vi "Refocus Frame v6 with morphology selection.vi"() -> ()   [LabVIEW 2018]
uses:
  <vilib>/Analysis/NI_AALBase.lvlib
  <vilib>/vision/NI_Vision_Development_Module.lvlib
panel:
  out "Number of Particles":i32
  in  "Use size  filter?":bool
  in  "Selection Values":T2(array[cluster]) {"Measurement Parameter" items=["Center of Mass X", "Center of Mass Y", "First Pixel X", "First Pixel Y", "Bounding Rect Left", "Bounding Rect Top", "Bounding Rect Right", "Bounding Rect Bottom", "Max Feret Diameter Start X", "Max Feret Diameter Start Y", "Max Feret Diameter End X", "Max Feret Diameter End Y", "Max Horiz. Segment Length Left", "Max Horiz. Segment Length Right", "Max Horiz. Segment Length Row", "-", "Bounding Rect Width", "Bounding Rect Height", "Bounding Rect Diagonal", "Perimeter", "Convex Hull Perimeter", "Holes' Perimeter", "Max Feret Diameter", "Equivalent Ellipse Major Axis", "Equivalent Ellipse Minor Axis", "Equivalent Ellipse Minor Axis (Feret)", "Equivalent Rect Long Side", "Equivalent Rect Short Side", "Equivalent Rect Diagonal", "Equivalent Rect Short Side (Feret)", "Average Horiz. Segment Length", "Average Vert. Segment Length", "Hydraulic Radius", "Waddel Disk Diameter", "-", "Area", "Holes' Area", "Particle & Holes' Area", "Convex Hull Area", "Image Area", "-", "Number of Holes", "Number of Horiz. Segments", "Number of Vert. Segments", "-", "Orientation", "Max Feret Diameter Orientation", "-", "% Area/Image Area", "% Area/(Particle & Holes' Area)", "Ratio of Equivalent Ellipse Axes", "Ratio of Equivalent Rect Sides", "-", "Elongation Factor", "Compactness Factor", "Heywood Circularity Factor", "Type Factor", "-", "Sum X", "Sum Y", "Sum XX", "Sum XY", "Sum YY", "Sum XXX", "Sum XXY", "Sum XYY", "Sum YYY", "-", "Moment of Inertia XX", "Moment of Inertia XY", "Moment of Inertia YY", "Moment of Inertia XXX", "Moment of Inertia XXY", "Moment of Inertia XYY", "Moment of Inertia YYY", "Norm. Moment of Inertia XX", "Norm. Moment of Inertia XY", "Norm. Moment of Inertia YY", "Norm. Moment of Inertia XXX", "Norm. Moment of Inertia XXY", "Norm. Moment of Inertia XYY", "Norm. Moment of Inertia YYY", "Hu Moment 1", "Hu Moment 2", "Hu Moment 3", "Hu Moment 4", "Hu Moment 5", "Hu Moment 6", "Hu Moment 7"]; "Range Lower Value" format="%.2f"; "Range Upper Value" format="%.2f"}
  in  "Decimate by N\n(even number!)":i32=1
  in  "Use image file as background?\n(N=> calculate from movie input)":bool=TRUE
  in  "Background image":path
  in  "Brightness (default = 1)":dbl=1.0
  out "Image":T3(plugin-control)
  in  "Threshold":dbl
  in  "Set threshold":bool
  in  "Number of frames for median":u32=20
  in  "Read Frame Number":u32
  in  "Input Movie":path
  in  "# parallel loops":i32=12
  in  "Write Gradient stack?":bool
  in  "Write Refocused stack?":bool=TRUE
  in  "Flip Z-gradient?":bool
  in  "Bandpass Filter?":bool=TRUE
  in  "Smallest object (px)":dbl=2.0
  in  "Largest object (px)":dbl=30.0
  out "Currently calculating \nrefocused frame number:":i32
  in  "Medium refractive index":dbl=1.3326
  in  "Pixels/micron":dbl=0.711
  in  "Wavelength (um)":dbl=0.642
  in  "Step size (um)":dbl=10.0
  in  "Number of steps":i32=150
  in  "Start refocus value (um)":dbl
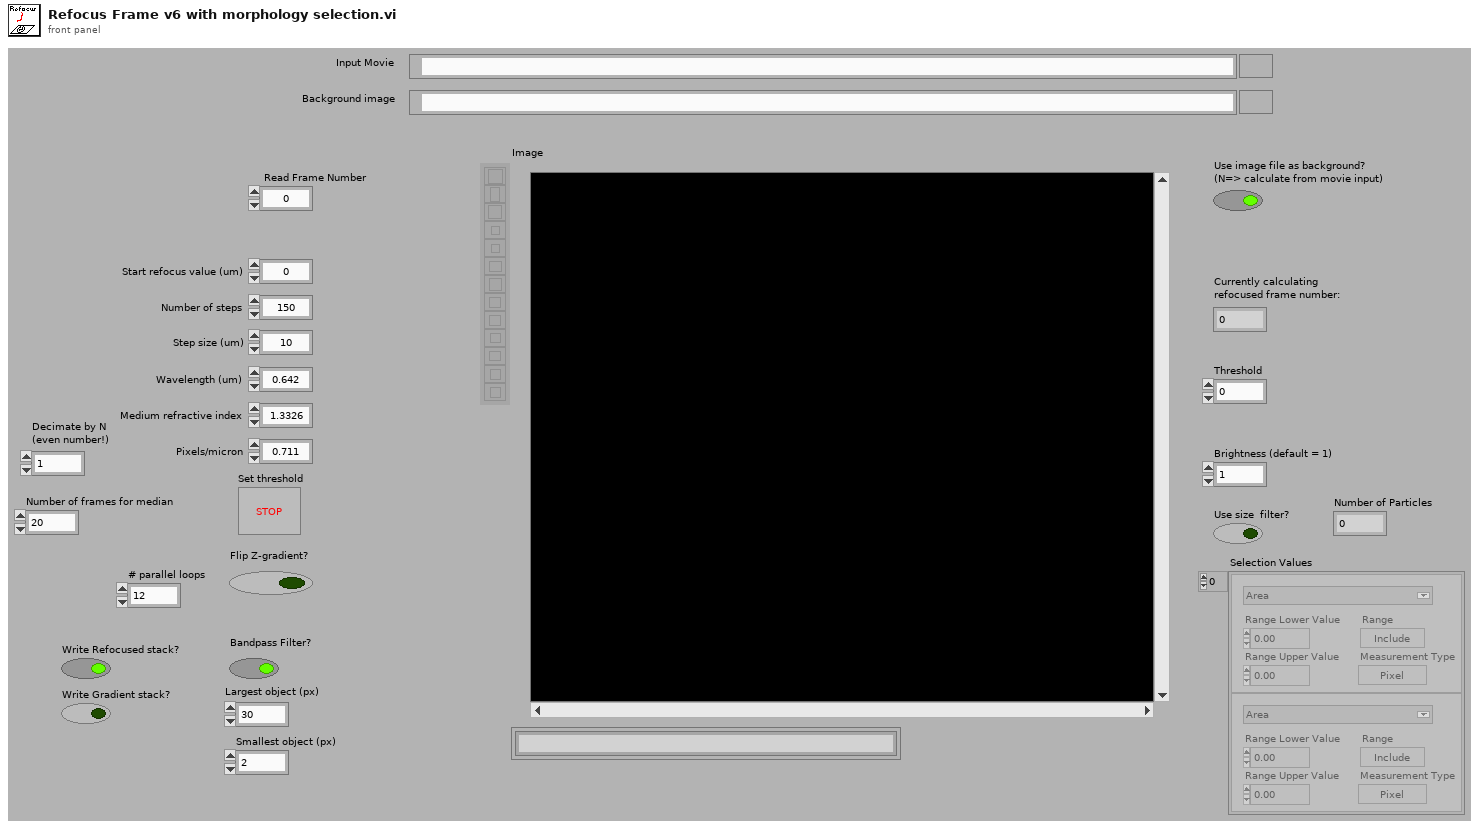
[diagram p1: front panel]
types:
  T1 = typedef "Particle Parameters" = i32
  T2 = cluster{"Measurement Parameter":T1, "Range Lower Value":dbl, "Range Upper Value":dbl, "Range":bool, "Measurement Type":bool}[]
  T3 = typedef "IMAQ Image.ctl" = refnum<image>
  T4 = typedef "Image Type" = u32
  T5 = typedef "AviRefnum.ctl" = refnum<k1>
  T6 = cluster{"Filter array":dbl[][], "Wavelength (um)":dbl, "Medium refractive index":dbl, dbl}
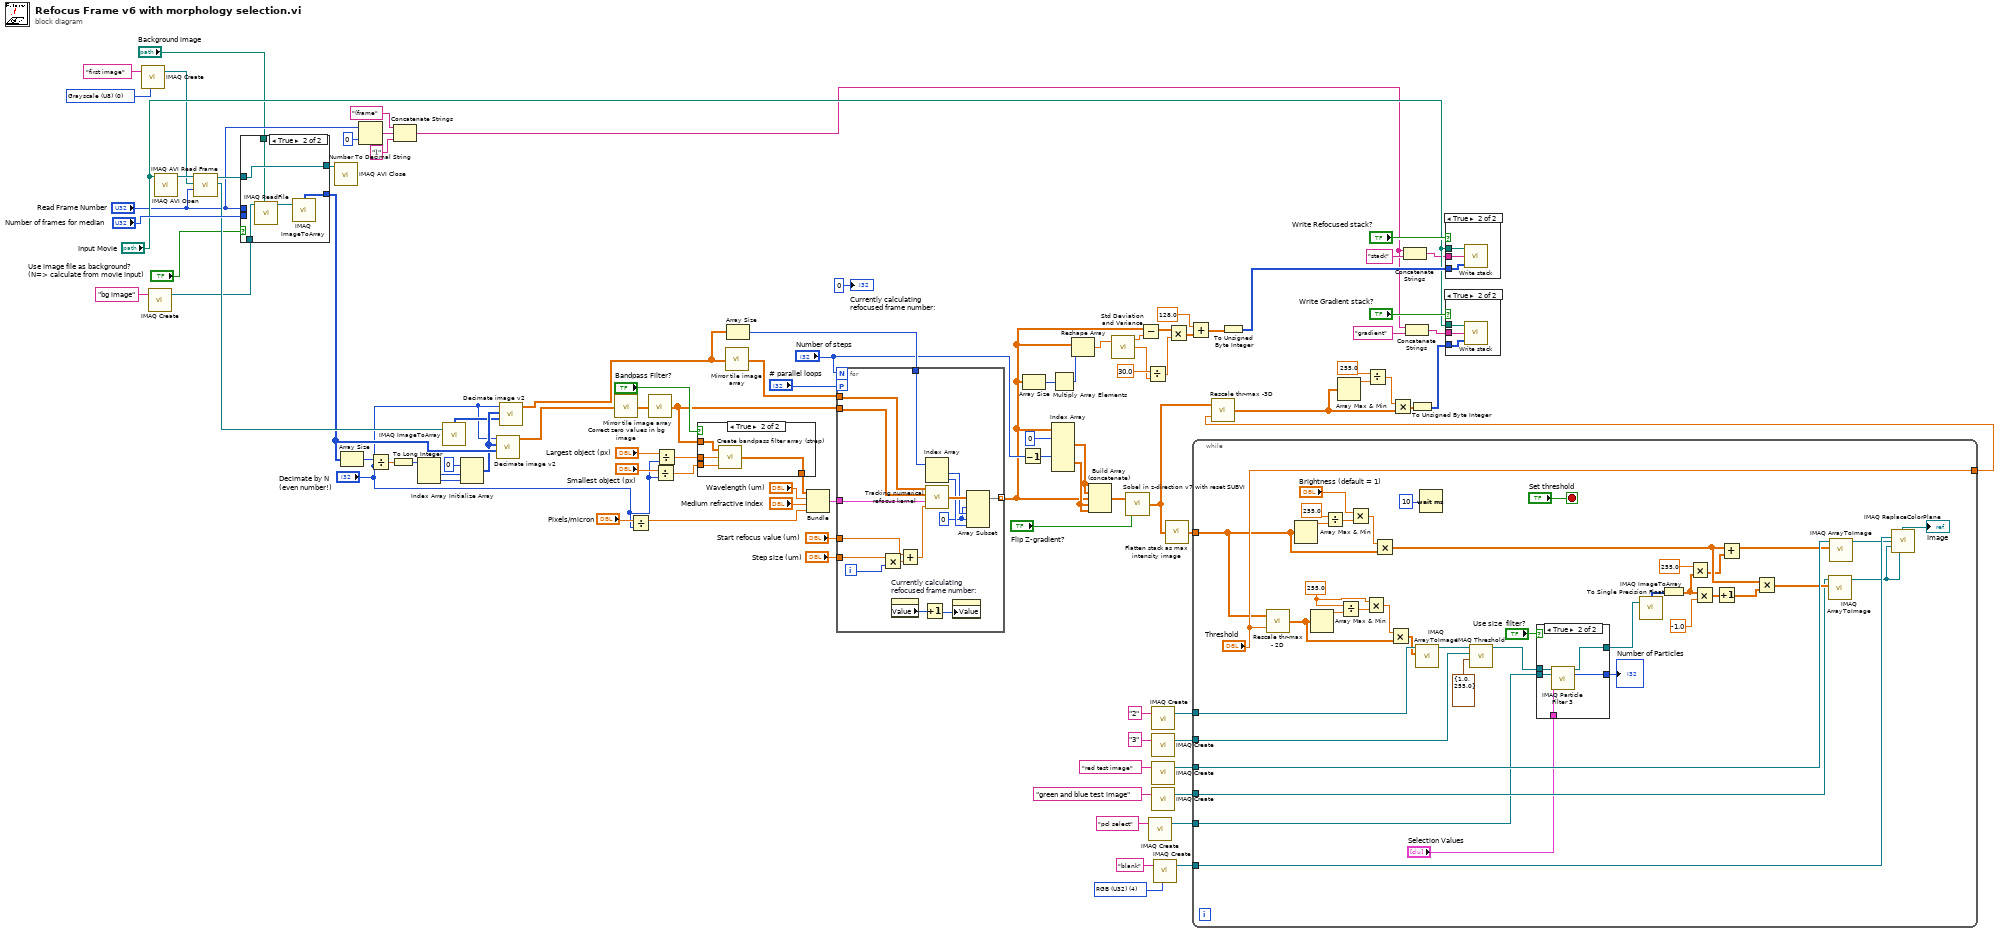
[diagram p0: block diagram]
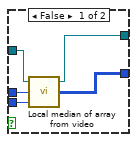
[diagram p2: hidden frame]
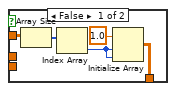
[diagram p6: hidden frame]
diagram:
  w3 = T4 4 items=["Grayscale (U8)", "Grayscale (I16)", "Grayscale (SGL)", "Complex (CSG)", "RGB (U32)", "HSL (U32)", "RGB (U64)", "Grayscale (U16)"] ("Image Type")
  w57 = T4 0 items=["Grayscale (U8)", "Grayscale (I16)", "Grayscale (SGL)", "Complex (CSG)", "RGB (U32)", "HSL (U32)", "RGB (U64)", "Grayscale (U16)"] ("Image Type")
  n1 = call "IMAQ Create"("Image Name"="first image", "Image Type"=w57) -> ("New Image"=w54:T3)  [unwired: 3 in, 1 out]
  n2 = call "IMAQ Create"("Image Name"="bg image") -> ("New Image"=w31:T3)  [unwired: 4 in, 1 out]
  n3 = call "IMAQ AVI Open"("AVI Path"="Input Movie") -> ("Avi Refnum"=w55:T5)  [unwired: 9 in, 1 out]
  n4 = call "IMAQ AVI Read Frame"("Frame Number"="Read Frame Number", "Image"=w54, "Avi Refnum"=w55) -> ("Image Out"=w53:T3, "Avi Refnum (duplicate)"=w52:T5)  [unwired: 5 in, 2 out]
  n5 = case shown="True" "Use image file as background?\n(N=> calculate from movie input)" {
    tunnel: "Number of frames for median" -> [w103 _]
    tunnel: w52 -> [w102 w108]
    tunnel: [w101 w108] -> w51
    tunnel: "Read Frame Number" -> [w100 _]
    tunnel: [w99 w104] -> w22
    tunnel: w31 -> [_ w106]
    tunnel: "Background image" -> [_ w105]
    frame False {
      n6 = call "Local median of array from video.vi"("Number of frames for median"=w103, "Read Frame Number"=w100, "Avi Refnum"=w102) -> ("Local median array"=w99:u8[][], "Avi Refnum (duplicate)"=w101:T5)  [unwired: 1 in]
    }
    frame True {
      n7 = call "IMAQ ReadFile"("File Path"=w105, "Image"=w106) -> ("Image Out"=w107:T3)  [unwired: 5 in, 4 out]
      n8 = call "IMAQ ImageToArray"("Image"=w107) -> ("Image Pixels (U8)"=w104:u8[][])  [unwired: 3 in, 4 out]
    }
  }
  n9 = call "IMAQ AVI Close"("Avi Refnum"=w51) -> ()  [unwired: 10 in, 1 out]
  n10 = Array Size(array=w22) -> (size(s)=w28:i32[])
  n11 = Number To Decimal String(number="Read Frame Number", width (-)=i16 0) -> (decimal integer string=w48:string)
  n12 = Divide(x=w28, y="Decimate by N\n(even number!)") -> (x/y=w27:dbl[])
  n13 = To Long Integer(number=w27) -> (32bit integer=w26:i32[])
  n14 = Concatenate Strings("(frame" ("string"), w48, ")" ("string")) -> (w42:string)
  n15 = Index Array(array=w26) -> (element #1=w25:i32, element #2=w24:i32)  [unwired: 2 in]
  n16 = call "IMAQ ImageToArray"("Image"=w53) -> ("Image Pixels (U8)"=w20:u8[][])  [unwired: 3 in, 4 out]
  n17 = Initialize Array(u8 0 ("element"), w25, w24) -> (w21:u8[][])
  n18 = call "Decimate image v2.vi"("Image Pixels (U8)"=w22, "Target array"=w21, "Decimate by N"="Decimate by N\n(even number!)") -> ("Filled target array"=w13:sgl[][])  [unwired: 8 in]
  n19 = call "Decimate image v2.vi"("Image Pixels (U8)"=w20, "Target array"=w21, "Decimate by N"="Decimate by N\n(even number!)") -> ("Filled target array"=w14:sgl[][])  [unwired: 8 in]
  n20 = call "Correct zero values in bg image.vi"("Image Pixels (U8)"=w13) -> ("Corrected array"=w83:sgl[][])
  n21 = Divide(x="Pixels/micron", y="Decimate by N\n(even number!)") -> (x/y=w19:dbl)
  n22 = call "Mirror tile image array.vi"("Image array"=w83) -> ("Mirror tiled array"=w81:sgl[][])
  n23 = Divide(x="Smallest object (px)", y="Decimate by N\n(even number!)") -> (x/y=w17:dbl)
  n24 = Divide(x="Largest object (px)", y="Decimate by N\n(even number!)") -> (x/y=w18:dbl)
  n25 = case shown="True" "Bandpass Filter?" {
    tunnel: w18 -> [_ w117]
    tunnel: w17 -> [_ w116]
    tunnel: w81 -> [w113 w115]
    tunnel: [w109 w114] -> w90
    frame False {
      n26 = Array Size(array=w113) -> (size(s)=w112:i32[])
      n27 = Index Array(array=w112) -> (element=w111:i32)  [unwired: 1 in]
      n28 = Initialize Array(1.0, w111, w111) -> (w109:dbl[][])
    }
    frame True {
      n29 = call "Create bandpass filter array (strep).vi"("Smallest object (pixels)"=w116, "Largest object (pixels)"=w117, "Image array"=w115) -> ("Filter array"=w114:dbl[][])
    }
  }
  n30 = call "Mirror tile image array.vi"("Image array"=w14) -> ("Mirror tiled array"=w84:sgl[][])
  n31 = Array Size(array=w14) -> (size(s)=w82:i32[])
  n32 = Bundle("Filter array"=w90, "Wavelength (um)"="Wavelength (um)", "Medium refractive index"="Medium refractive index", w19) -> (w92:T6)  [unwired: 1 in]
  n33 = for {
    N: "Number of steps" -> [_]
    tunnel: "Start refocus value (um)" -> [w131]
    tunnel: "Step size (um)" -> [w133]
    tunnel: w81 -> [w129]
    tunnel: [w125] -> w60 mode=indexing
    tunnel: w92 -> [w128]
    tunnel: w84 -> [w127]
    tunnel: w82 -> [w124]
    workers-P: "# parallel loops" -> [_]
    i -> [w120]
    w121 = 0 ("x+1")
    n34 = Multiply(x=w133, y=w120) -> (x*y=w132:dbl)
    n35 = property on="Currently calculating \nrefocused frame number:" class="DigNum (strict)"() -> ("Value"=w118:i32)  [unwired: 2 in, 2 out]
    n36 = Add(x=w131, y=w132) -> (x+y=w130:dbl)
    n37 = Increment(x=w118) -> (x+1=w119:i32)
    n38 = Index Array(array=w124) -> (element #1=w123:i32, element #2=w122:i32)  [unwired: 2 in]
    n39 = call "Tracking numerical refocus kernel.vi"("Defocus distance (um)"=w130, "Control Cluster"=w128, "Corrected array"=w129, "Image array"=w127) -> ("output array"=w126:dbl[][])
    n40 = property on="Currently calculating \nrefocused frame number:" class="DigNum (strict)"("Value"=w119) -> ()  [unwired: 2 in, 2 out]
    n41 = Array Subset(array=w126, index (row)=w121, length (row)=w123, index (col)=w121, length (col)=w122) -> (w125:dbl[][])
  }
  n42 = Decrement(x="Number of steps") -> (x-1=w74:i32)
  n43 = Array Size(array=w60) -> (size(s)=w61:i32[])
  n44 = Index Array(array=w60, index (dim 0) #1=0 ("x+1"), index (dim 0) #2=w74) -> (element #1=w73:dbl[][], element #2=w72:dbl[][])  [unwired: 4 in]
  n45 = Multiply Array Elements(1:w61) -> (0:w59:i32)
  n46 = Reshape Array(w60, w59) -> (w50:dbl[])
  n47 = Build Array (concatenate)(w73, w73, w60, w72, w72) -> (w71:dbl[][][])
  n48 = call <vilib>:"Std Deviation and Variance.vi"("X"=w50) -> ("mean"=w70:dbl, "standard deviation"=w68:dbl)  [unwired: 1 in, 1 out]
  n49 = call "Sobel in z-direction v7 with reset SUBVI.vi"("Flip Z-gradient?"="Flip Z-gradient?", "Recontructed Stack\n(with padded ends)"=w71) -> ("Sobel output stack"=w6:dbl[][][])
  n50 = Subtract(x=w60, y=w70) -> (x-y=w67:dbl[][][])
  n51 = Divide(x=30.0 ("Start refocus value (um)"), y=w68) -> (x/y=w66:dbl)
  n52 = call "IMAQ Create"("Image Name"="pcl select") -> ("New Image"=w1:T3)  [unwired: 4 in, 1 out]
  n53 = call "IMAQ Create"("Image Name"="2") -> ("New Image"=w11:T3)  [unwired: 4 in, 1 out]
  n54 = call "IMAQ Create"("Image Name"="3") -> ("New Image"=w9:T3)  [unwired: 4 in, 1 out]
  n55 = call "IMAQ Create"("Image Name"="red test image") -> ("New Image"=w38:T3)  [unwired: 4 in, 1 out]
  n56 = call "IMAQ Create"("Image Name"="green and blue test image") -> ("New Image"=w7:T3)  [unwired: 4 in, 1 out]
  n57 = call "IMAQ Create"("Image Name"="blank", "Image Type"=w3) -> ("New Image"=w4:T3)  [unwired: 3 in, 1 out]
  n58 = call "Flatten stack as max intensity image.vi"("Input image stack"=w6) -> ("Max intensity 2D array"=w39:sgl[][])
  n59 = Multiply(x=w67, y=w66) -> (x*y=w64:dbl[][][])
  n60 = Add(x=128.0 ("Start refocus value (um)"), y=w64) -> (x+y=w65:dbl[][][])
  n61 = while {
    tunnel: w39 -> [w165]
    tunnel: w38 -> [w173]
    tunnel: ["Threshold"] -> w37
    tunnel: w11 -> [w160]
    tunnel: w9 -> [w157]
    tunnel: w7 -> [w150]
    tunnel: w4 -> [w148]
    tunnel: w1 -> [w139]
    stop <- "Set threshold" stop-if-true
    w155 = 255.0 ("x+1")
    n62 = call "Rescale thr-max - 2D.vi"("Threshold"="Threshold", "Max intensity 2D array"=w165) -> ("Thresholded Array"=w161:dbl[][])
    n63 = Array Max & Min(array=w165) -> (max value=w171:sgl)  [unwired: 3 out]
    n64 = Array Max & Min(array=w161) -> (max value=w164:dbl)  [unwired: 3 out]
    n65 = Divide(x=255.0 ("x+1"), y=w171) -> (x/y=w169:dbl)
    n66 = Divide(x=w155, y=w164) -> (x/y=w163:dbl)
    n67 = Multiply(x="Brightness (default = 1)", y=w169) -> (x*y=w167:dbl)
    n68 = Multiply(x=w155, y=w163) -> (x*y=w162:dbl)
    n69 = Multiply(x=w167, y=w165) -> (x*y=w152:dbl[][])
    n70 = Multiply(x=w162, y=w161) -> (x*y=w159:dbl[][])
    n71 = call "IMAQ ArrayToImage"("Image Pixels (U8)"=w159, "Image"=w160) -> ("Image Out"=w158:T3)  [unwired: 8 in, 1 out]
    n72 = Wait (ms)(milliseconds to wait=u32 10) -> ()  [unwired: 1 out]
    n73 = call "IMAQ Threshold"("Range"=cluster{"Lower value":sgl, "Upper value":sgl} {"Lower value"=1.0, "Upper value"=255.0}, "Image Dst"=w157, "Image Src"=w158) -> ("Image Dst Out"=w137:T3)  [unwired: 7 in, 1 out]
    n74 = case shown="True" "Use size  filter?" {
      tunnel: w139 -> [_ w180]
      tunnel: "Selection Values" -> [_ w179]
      tunnel: w137 -> [w175 w178]
      tunnel: [w175 w177] -> w136
      tunnel: [_ w176] -> w134
      frame False {
      }
      frame True {
        n75 = call "IMAQ Particle Filter 3"("Image Src"=w178, "Image Dst"=w180, "Selection Values"=w179) -> ("Image Dst Out"=w177:T3, "Number of Particles"=w176:i32)  [unwired: 10 in, 1 out]
      }
    }
    "Number of Particles" <- w134
    n76 = call "IMAQ ImageToArray"("Image"=w136) -> ("Image Pixels (U8)"=w154:u8[][])  [unwired: 3 in, 4 out]
    n77 = To Single Precision Float(number=w154) -> (single precision float=w143:sgl[][])
    n78 = Multiply(x=255.0 ("x+1"), y=w143) -> (x*y=w145:dbl[][])
    n79 = Multiply(x=w143, y=-1.0 ("x+1")) -> (x*y=w141:dbl[][])
    n80 = Increment(x=w141) -> (x+1=w140:dbl[][])
    n81 = Add(x=w152, y=w145) -> (x+y=w146:dbl[][])
    n82 = Multiply(x=w152, y=w140) -> (x*y=w151:dbl[][])
    n83 = call "IMAQ ArrayToImage"("Image Pixels (U8)"=w151, "Image"=w150) -> ("Image Out"=w144:T3)  [unwired: 8 in, 1 out]
    n84 = call "IMAQ ArrayToImage"("Image Pixels (U8)"=w146, "Image"=w173) -> ("Image Out"=w147:T3)  [unwired: 8 in, 1 out]
    n85 = call "IMAQ ReplaceColorPlane"("Image Dst"=w148, "Red or Hue Plane"=w147, "Green or Sat Plane"=w144, "Blue or Luma or Val or Inten Plane"=w144) -> ("Image Dst Out"=→"Image":T3)  [unwired: 10 in, 1 out]
  }
  n86 = call "Rescale thr-max -3D.vi"("Threshold"=w37, "3D array"=w6) -> ("Thresholded Array"=w33:dbl[][][])
  n87 = To Unsigned Byte Integer(number=w65) -> (unsigned 8bit integer=w78:u8[][][])
  n88 = Array Max & Min(array=w33) -> (max value=w36:dbl)  [unwired: 3 out]
  n89 = Divide(x=255.0 ("x+1"), y=w36) -> (x/y=w34:dbl)
  n90 = Multiply(x=w34, y=w33) -> (x*y=w41:dbl[][][])
  n91 = Concatenate Strings(w42, "stack" ("Image Name")) -> (w44:string)
  n92 = Concatenate Strings(w42, "gradient" ("Image Name")) -> (w43:string)
  n93 = To Unsigned Byte Integer(number=w41) -> (unsigned 8bit integer=w62:u8[][][])
  n94 = case shown="True" "Write Refocused stack?" {
    tunnel: w44 -> [_ w183]
    tunnel: w78 -> [_ w182]
    tunnel: "Input Movie" -> [_ w181]
    frame False {
    }
    frame True {
      n95 = call "Write stack.vi"("Normalised array"=w182, "Image buffer name"=w183, "Input image path"=w181) -> ()
    }
  }
  n96 = case shown="True" "Write Gradient stack?" {
    tunnel: w43 -> [_ w186]
    tunnel: w62 -> [_ w185]
    tunnel: "Input Movie" -> [_ w184]
    frame False {
    }
    frame True {
      n97 = call "Write stack.vi"("Normalised array"=w185, "Image buffer name"=w186, "Input image path"=w184) -> ()
    }
  }
  "Currently calculating \nrefocused frame number:" <- 0 ("Currently calculating \nrefocused frame number:")
